vi "tm_getrecorderstatus.vi"(8 "error in (no error)":errorcluster, 11 "Handle":u32) -> (0 "error out":errorcluster, 1 "Count":i32, 2 "Index":i32, 3 "Handle":u32)   [LabVIEW 2023]
uses:
  tmcamcon.dll
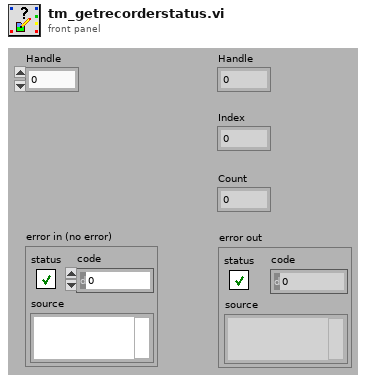
[diagram p1: front panel]
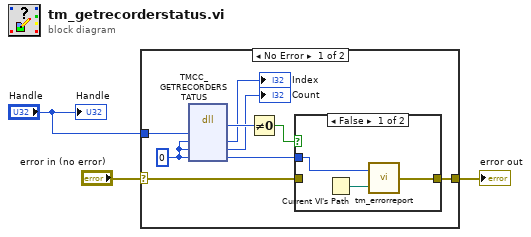
[diagram p0: block diagram]
diagram:
  n1 = case shown="No Error" "error in (no error)" {
    selector: "error in (no error)" -> [w8 w17]
    tunnel: [w4 w17] -> w2
    tunnel: "Handle" -> [w11 _]
    frame No Error {
      w5 = 0
      n2 = dll-call lib="tmcamcon.dll" fn="TMCC_GETRECORDERSTATUS"("handle"=w11, "index"=w5, "count"=w5, "Erval"=w5) -> ("return type"=w12:u32, "index"=→"Index":i32, "count"=→"Count":i32, "Erval"=w7:i32)  [unwired: 4 in, 2 out]
      n3 = Not Equal To 0?(x=w12) -> (x != 0?=w6:bool)
      n4 = case shown="False" w6 {
        tunnel: w8 -> [_ w16]
        tunnel: [w14 w16] -> w4
        tunnel: w7 -> [w13 _]
        frame False {
          n5 = Current VI's Path() -> (path=w15:path)
          n6 = call "tm_errorreport.vi"("Source"=w15, "Error"=w13) -> ("error out"=w14:errorcluster)
        }
        frame True {
        }
      }
    }
    frame Error {
    }
  }
  "error out" <- w2
  "Handle" <- "Handle"
